vi "GV line count.vi"() -> ()   [LabVIEW 2017]
panel:
  out "Line count":u16
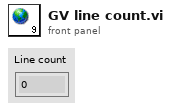
[diagram p1: front panel]
diagram:
